vi "ResultData_SM.vi"(8 "error in (no error)":errorcluster, 10 "Result Cluster":T1, 11 "Inspection Statemachine in":refnum<class "Inspection Statemachine.lvclass">) -> (0 "error out":errorcluster, 3 "Inspection Statemachine out":refnum<class "Inspection Statemachine.lvclass">)   [LabVIEW 2019, in "Inspection Statemachine.lvclass"]
uses:
  Inspection Statemachine.lvclass
  <vilib>/vision/Image Controls.llb/IMAQ Image.ctl
  Controls/Result Cluster_SM.ctl
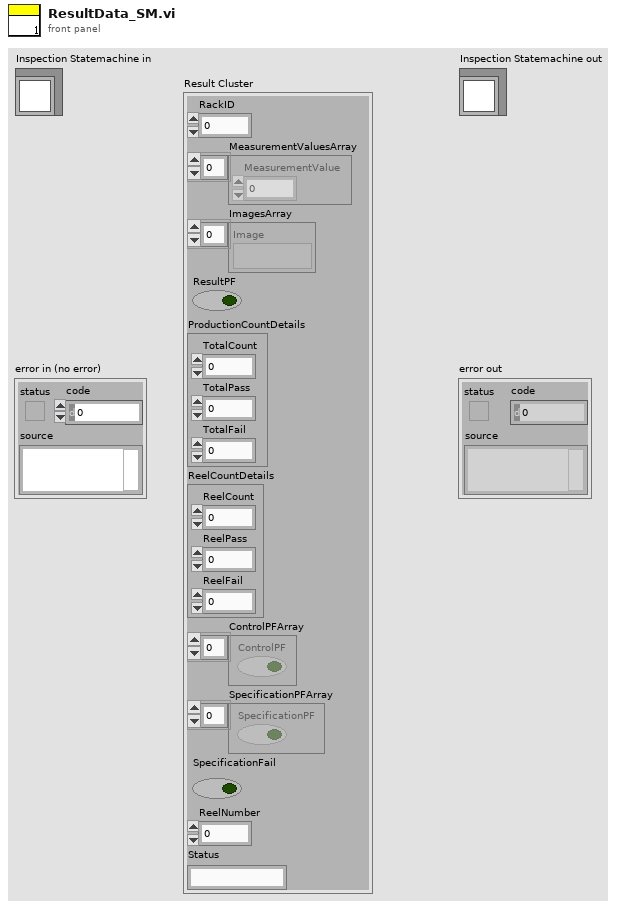
[diagram p1: front panel]
types:
  T1 = typedef "Inspection Statemachine.lvclass/Result Cluster_SM.ctl" = cluster{"RackID":u8, "MeasurementValuesArray ":dbl[], "ImagesArray":T2[], "ResultPF":bool, "ProductionCountDetails":cluster{"TotalFail":u64, "TotalPass":u64, "TotalCount":u64}, "ReelCountDetails":cluster{"ReelFail":u64, "ReelPass":u64, "ReelCount":u64}, "ControlPFArray":bool[], "SpecificationPFArray":bool[], "SpecificationFail":bool, "ReelNumber":u64, "Status":string}
  T2 = typedef "IMAQ Image.ctl" = refnum<image>
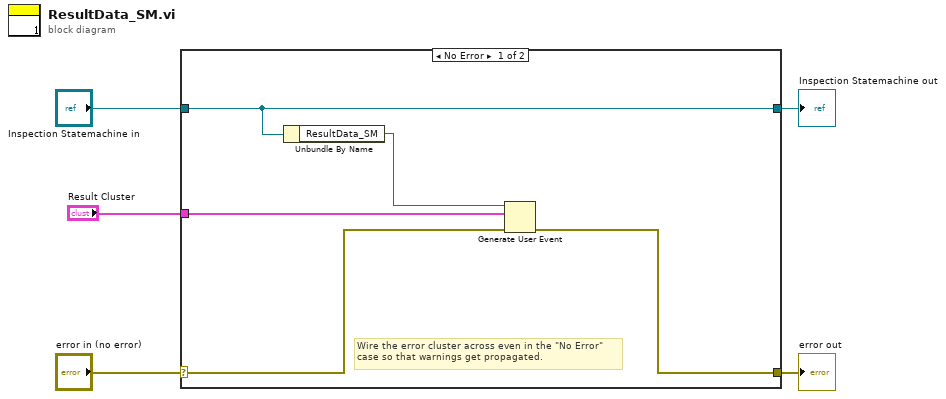
[diagram p0: block diagram]
diagram:
  n1 = case shown="No Error" "error in (no error)" {
    selector: "error in (no error)" -> [w10 w12]
    tunnel: [w9 w12] -> w4
    tunnel: [w8 w11] -> w2
    tunnel: "Inspection Statemachine in" -> [w8 w11]
    tunnel: "Result Cluster" -> [w6 _]
    frame No Error {
      # "Wire the error cluster across even in the \"No Error\"\ncase so that warnings get propagated."
      n2 = Unbundle By Name(w8) -> ("ResultData_SM"=w7:refnum<user-event>)
      n3 = Generate User Event(user event=w7, event data cluster=w6, error in=w10) -> (error out=w9:errorcluster)  [unwired: 1 in, 1 out]
    }
    frame Error {
    }
  }
  "error out" <- w4
  "Inspection Statemachine out" <- w2
